vi "Auto_Drive.vi"(8 "Timer?":bool, 9 "Duration":u32=3500, 10 "distance":dbl=88.0 format="%#_13g", 11 "Drive Effort":dbl=1000.0) -> ()   [LabVIEW 2016]
uses:
  <vilib>/Rock Robotics/WPI/SafetyOutput/WPI_SafetyOutputConfigMenu.ctl
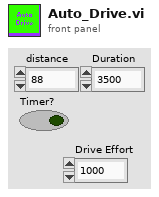
[diagram p1: front panel]
types:
  T1 = typedef "WPI_SafetyOutputConfigMenu.ctl" = enum16{"Enable", "Disable"}
  T2 = typedef "WPI_MotorControlDeviceRef.ctl" = cluster{"DeviceStatus":errorcluster, "Type":T3, "PWM":cluster{"PWM Channel":T4, "DeadBand":T5}, "CAN":cluster{"Device Number":u8, "SetOutput VI Ref":variant, "GetOutput VI Ref":variant, "Enable VI Ref":variant, "Disable VI Ref":variant, "Data":variant}, "Invert":bool}
  T3 = typedef "WPI_MotorControlType.ctl" = enum16{"PWM", "CAN"}
  T4 = typedef "FPGA_DIOPWMChannel.ctl" = enum8{"PWM 0", "PWM 1", "PWM 2", "PWM 3", "PWM 4", "PWM 5", "PWM 6", "PWM 7", "PWM 8", "PWM 9", "PWM MXP 0", "PWM MXP 1", "PWM MXP 2", "PWM MXP 3", "PWM MXP 4", "PWM MXP 5", "PWM MXP 6", "PWM MXP 7", "PWM MXP 8", "PWM MXP 9", "Invalid"}
  T5 = typedef "WPI_PWMDeadband.ctl" = cluster{"Name":string, "maxPositivePwm":i32, "minPositivePwm":i32, "centerPwm":i32, "maxNegativePwm":i32, "minNegativePwm":i32, "angularRange":u16}
  T6 = typedef "WPI_CANTalonSRX_GlobalStatus.ctl" = cluster{"Applied Throttle":dbl, "Module Enabled":bool, "CAN Error":errorcluster, "Closed Loop Error":dbl, "Forward Limit Switch Closed":bool, "Reverse Limit Switch Closed":bool, "Sensor Position":dbl, "Sensor Velocity":dbl, "Current":dbl, "Sticky Fault - Over Temp":bool, "Sticky Fault - Under Voltage":bool, "Sticky Fault - Forward Limit":bool, "Sticky Fault - Reverse Limit":bool, "Sticky Fault - Forward Soft Limit":bool, "Sticky Fault - Reverse Soft Limit":bool, "Brake is Enabled":bool, "Encoder Position":dbl, "Encoder Velocity":dbl, "Encoder Index Count":dbl, "Encoder A Pin State":bool, "Encoder B Pin State":bool, "Encoder Index Pin State":bool, "Analog In":dbl, "Analog In Velocity":dbl, "Temperature (C)":dbl, "Battery Voltage":dbl, "Control 5 Is Supported":bool, "Current Profile Slot Select":dbl, "Pos Div 8":bool, "Vel Div 4":bool, "Pulse Width Position":i32, "Pulse Width Velocity":i32, "Pulse Width Rise To Rise (us)":i32, "Pulse Width Rise To Fall (us)":i32, "Mot Prof Active Is Under Run":bool, "Mot Prof Active Has Under Run":bool, "Mot Prof Active Is Last":bool, "Mot Prof Active Velocity Only":bool, "Mot Prof Active Is Valid":bool, "Mot Prof Buffer Is Full":bool, "Mot Prof Active Profile Slot Select":i32, "Mot Prof NextID":i32, "Mot Prof Count":i32, "Mot Prof Active Velocity":dbl, "Mot Prof Active Position":dbl, "Mot Prof Output Enable":i32}
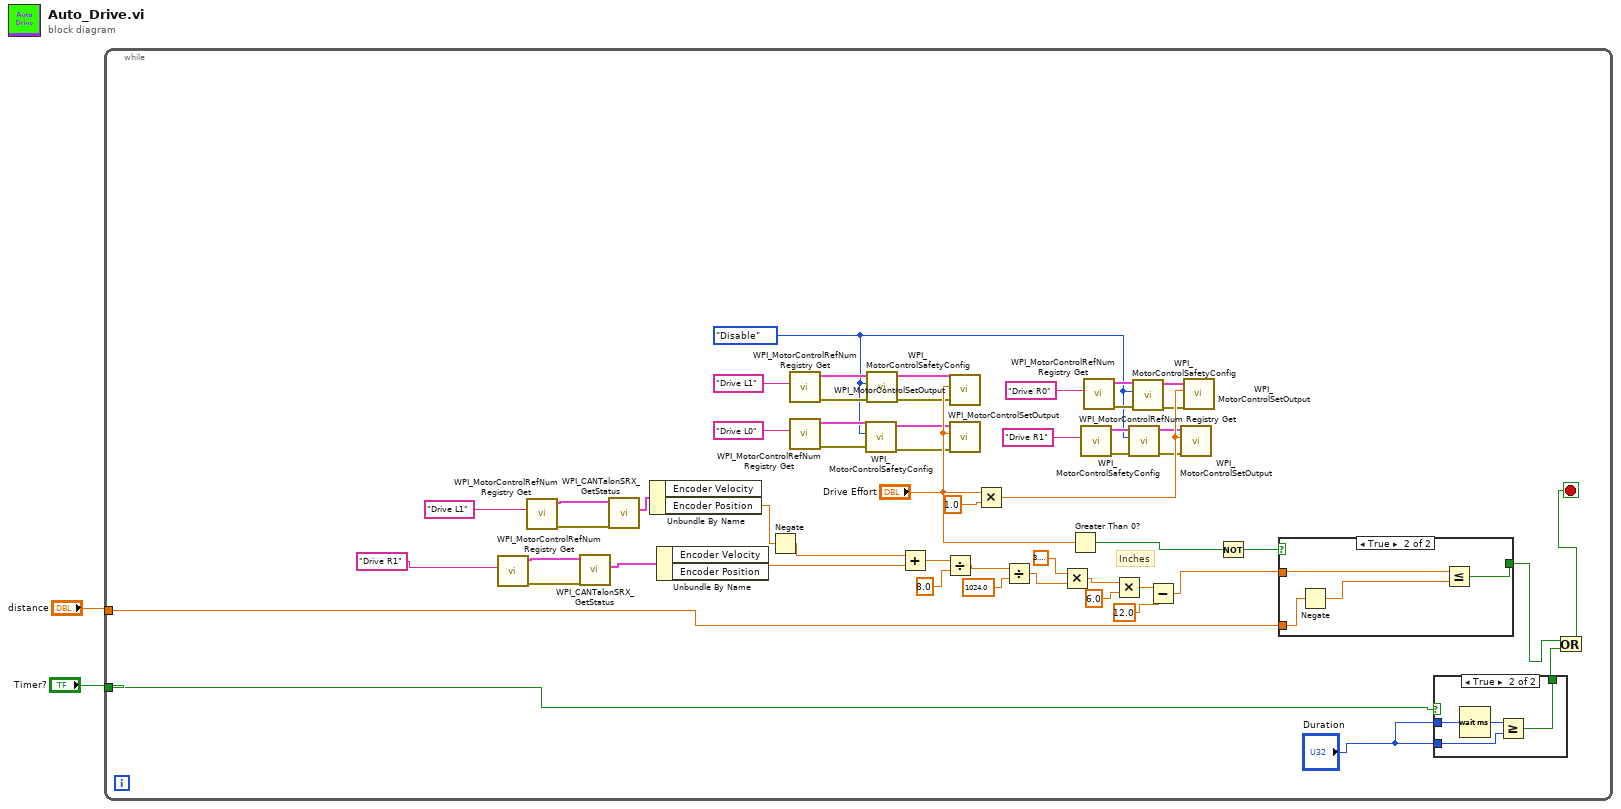
[diagram p0: block diagram]
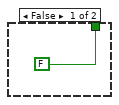
[diagram p2: hidden frame]
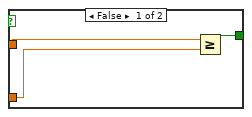
[diagram p3: hidden frame]
diagram:
  n1 = while {
    tunnel: "distance" -> [w35]
    tunnel: "Timer?" -> [w30]
    stop <- w24 stop-if-true
    w3 = WPI_SafetyOutputConfigMenu."Disable" ("mode")
    # "Inches"
    n2 = call <vilib>:"WPI_MotorControlRefNum Registry Get.vi"("refnum name"="Drive R1") -> ("error out"=w52:errorcluster, "MotorControlDevRef"=w53:T2)  [unwired: 9 in]
    n3 = call <vilib>:"WPI_MotorControlRefNum Registry Get.vi"("refnum name"="Drive L1") -> ("error out"=w49:errorcluster, "MotorControlDevRef"=w54:T2)  [unwired: 9 in]
    n4 = call <vilib>:"WPI_CANTalonSRX_GetStatus.vi"("error in (no error)"=w52, "CAN Talon SRX Ref"=w53) -> ("Talon SRX Status"=w50:T6)  [unwired: 7 in, 2 out]
    n5 = call <vilib>:"WPI_CANTalonSRX_GetStatus.vi"("error in (no error)"=w49, "CAN Talon SRX Ref"=w54) -> ("Talon SRX Status"=w51:T6)  [unwired: 7 in, 2 out]
    n6 = Unbundle By Name(w51) -> ("Encoder Position"=w48:dbl)  [unwired: 1 out]
    n7 = Unbundle By Name(w50) -> ("Encoder Position"=w38:dbl)  [unwired: 1 out]
    n8 = Negate(x=w48) -> (-x=w47:dbl)
    n9 = call <vilib>:"WPI_MotorControlRefNum Registry Get.vi"("refnum name"="Drive L1") -> ("error out"=w18:errorcluster, "MotorControlDevRef"=w19:T2)  [unwired: 9 in]
    n10 = call <vilib>:"WPI_MotorControlRefNum Registry Get.vi"("refnum name"="Drive L0") -> ("error out"=w14:errorcluster, "MotorControlDevRef"=w15:T2)  [unwired: 9 in]
    n11 = call <vilib>:"WPI_MotorControlSafetyConfig.vi"("error in (no error)"=w14, "mode"=w3, "MotorControlDevRef"=w15) -> ("error out"=w12:errorcluster, "MotorControlDevRef"=w13:T2)  [unwired: 7 in]
    n12 = call <vilib>:"WPI_MotorControlSafetyConfig.vi"("error in (no error)"=w18, "mode"=w3, "MotorControlDevRef"=w19) -> ("error out"=w16:errorcluster, "MotorControlDevRef"=w17:T2)  [unwired: 7 in]
    n13 = Add(x=w47, y=w38) -> (x+y=w46:dbl)
    n14 = Divide(x=w46, y=8.0) -> (x/y=w44:dbl)
    n15 = call <vilib>:"WPI_MotorControlSetOutput.vi"("error in (no error)"=w16, "Output"="Drive Effort", "MotorControlDevRef"=w17) -> ()  [unwired: 6 in, 3 out]
    n16 = call <vilib>:"WPI_MotorControlSetOutput.vi"("error in (no error)"=w12, "Output"="Drive Effort", "MotorControlDevRef"=w13) -> ()  [unwired: 6 in, 3 out]
    n17 = Multiply(x="Drive Effort", y=1.0) -> (x*y=w21:dbl)
    n18 = Divide(x=w44, y=1024.0) -> (x/y=w42:dbl)
    n19 = Multiply(x=3.141592653589793, y=w42) -> (x*y=w40:dbl)
    n20 = Greater Than 0?(x="Drive Effort") -> (x > 0?=w31:bool)
    n21 = call <vilib>:"WPI_MotorControlRefNum Registry Get.vi"("refnum name"="Drive R1") -> ("error out"=w6:errorcluster, "MotorControlDevRef"=w7:T2)  [unwired: 9 in]
    n22 = call <vilib>:"WPI_MotorControlRefNum Registry Get.vi"("refnum name"="Drive R0") -> ("error out"=w10:errorcluster, "MotorControlDevRef"=w11:T2)  [unwired: 9 in]
    n23 = Multiply(x=w40, y=6.0) -> (x*y=w34:dbl)
    n24 = call <vilib>:"WPI_MotorControlSafetyConfig.vi"("error in (no error)"=w6, "mode"=w3, "MotorControlDevRef"=w7) -> ("error out"=w5:errorcluster, "MotorControlDevRef"=w4:T2)  [unwired: 7 in]
    n25 = call <vilib>:"WPI_MotorControlSafetyConfig.vi"("error in (no error)"=w10, "mode"=w3, "MotorControlDevRef"=w11) -> ("error out"=w9:errorcluster, "MotorControlDevRef"=w8:T2)  [unwired: 7 in]
    n26 = Subtract(x=w34, y=12.0) -> (x-y=w32:dbl)
    n27 = call <vilib>:"WPI_MotorControlSetOutput.vi"("error in (no error)"=w5, "Output"=w21, "MotorControlDevRef"=w4) -> ()  [unwired: 6 in, 3 out]
    n28 = call <vilib>:"WPI_MotorControlSetOutput.vi"("error in (no error)"=w9, "Output"=w21, "MotorControlDevRef"=w8) -> ()  [unwired: 6 in, 3 out]
    n29 = Not(x=w31) -> (.not. x?=w22:bool)
    n30 = case shown="True" w22 {
      tunnel: [w62 w68] -> w26
      tunnel: w35 -> [w63 w66]
      tunnel: w32 -> [w64 w65]
      frame False {
        n31 = Greater Or Equal?(x=w64, y=w63) -> (x >= y?=w62:bool)
      }
      frame True {
        n32 = Negate(x=w66) -> (-x=w67:dbl)
        n33 = Less Or Equal?(x=w65, y=w67) -> (x <= y?=w68:bool)
      }
    }
    n34 = case shown="True" w30 {
      tunnel: "Duration" -> [_ w60]
      tunnel: [FALSE w59] -> w25
      tunnel: "Duration" -> [_ w58]
      frame False {
      }
      frame True {
        n35 = Wait (ms)(milliseconds to wait=w58) -> (millisecond timer value=w61:u32)
        n36 = Greater Or Equal?(x=w61, y=w60) -> (x >= y?=w59:bool)
      }
    }
    n37 = Or(x=w26, y=w25) -> (x .or. y?=w24:bool)
  }
